vi "calculate_image_indexes.vi"(4 "error in":errorcluster, 6 "y":i32=512, 7 "x":i32=512) -> (0 "error out":errorcluster, 3 "RGB index":i32[](array[numeric]))   [LabVIEW 2019]
doc: "Calculate the indexes of interes on the RGBA array to obtain a RGB array."
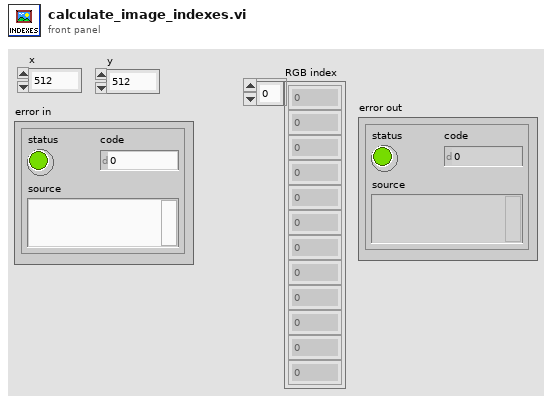
[diagram p1: front panel]
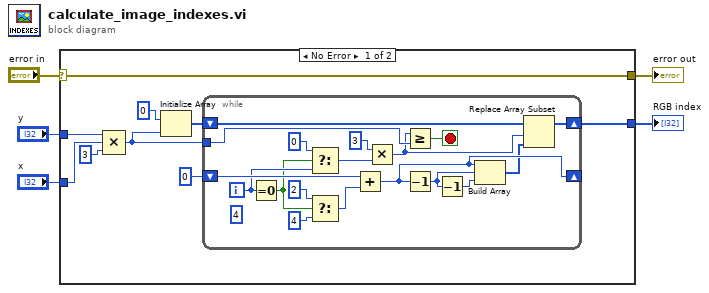
[diagram p0: block diagram]
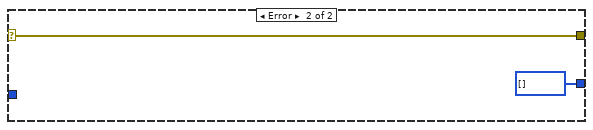
[diagram p2: hidden frame]
diagram:
  n1 = case shown="No Error" "error in" {
    selector: "error in" -> [w6 w33]
    tunnel: "y" -> [w14 _]
    tunnel: "x" -> [w13 _]
    tunnel: [w7 i32[] []] -> w3
    tunnel: [w6 w33] -> w2
    frame No Error {
      n2 = Compound Arithmetic op=MULTIPLY(w14, w13, 3 ("value")) -> (w11:i32)
      n3 = Initialize Array(0, w11) -> (w8:i32[])
      n4 = while {
        shift-right: [w30] -> w7
        shift-left: w8 -> [w31]
        tunnel: w11 -> [w29]
        shift-right: [w25] -> _
        shift-left: 0 ("index") -> [w26]
        i -> [w21]
        stop <- w32 stop-if-true
        (unwired) 4 ("y")
        n5 = Equal To 0?(x=w21) -> (x = 0?=w20:bool)
        n6 = Select(t=0, s=w20, f=w21) -> (s? t:f=w16:i32)
        n7 = Select(t=2, s=w20, f=4 ("y")) -> (s? t:f=w15:i32)
        n8 = Add(x=w26, y=w15) -> (x+y=w25:i32)
        n9 = Multiply(x=3, y=w16) -> (x*y=w28:i32)
        n10 = Greater Or Equal?(x=w28, y=w29) -> (x >= y?=w32:bool)
        n11 = Decrement(x=w25) -> (x-1=w22:i32)
        n12 = Decrement(x=w22) -> (x-1=w24:i32)
        n13 = Build Array(w25, w22, w24) -> (w23:i32[])
        n14 = Replace Array Subset(array=w31, new element=w23, index=w28) -> (w30:i32[])
      }
    }
    frame Error {
    }
  }
  "error out" <- w2
  "RGB index" <- w3
